vi "Read Config.vi"(8 "error in (no error)":errorcluster, 11 "Path":path) -> (0 "error out":errorcluster, 2 "Config":T1, 3 "File Created?":bool)   [LabVIEW 2020, in "VI Properties Editor.lvlib"]
doc: "Reads a config file located at <B>Path</B>."
uses:
  VI Properties Editor.lvlib
  CTLs/Config.ctl
  CTLs/Filter Info.ctl
  CTLs/Filter Column.ctl
  CTLs/Filter Type.ctl
  CTLs/Config Key.ctl
  9b94a6d9-a102-4d4c-a75a-250a13817fae.vi
  <vilib>/Utility/config.llb/Read Key (U32).vi
  <vilib>/Utility/config.llb/Read Key (String).vi
  <vilib>/Utility/config.llb/Read Key (Boolean).vi
  <vilib>/Utility/config.llb/Read Key (I32).vi
  <vilib>/Utility/config.llb/NI_LVConfig.lvlib
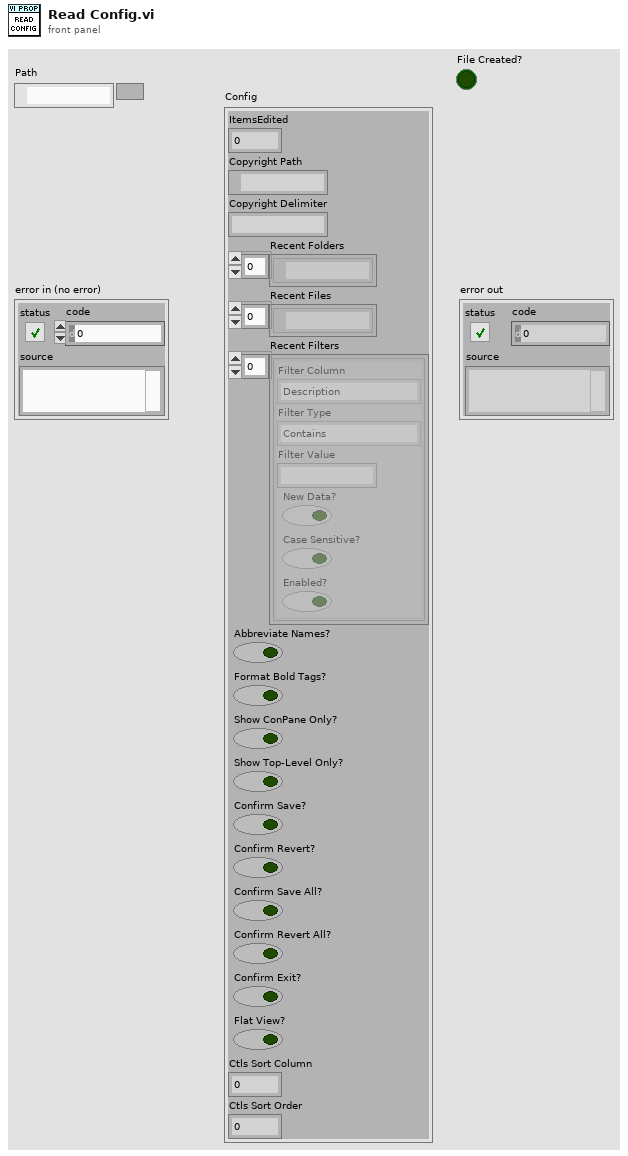
[diagram p1: front panel]
types:
  T1 = typedef "VI Properties Editor.lvlib/Config.ctl" = cluster{"ItemsEdited":u32, "Copyright Path":path, "Copyright Delimiter":string, "Recent Folders":path[], "Recent Files":path[], "Recent Filters":T2[], "Abbreviate Names?":bool, "Format Bold Tags?":bool, "Show ConPane Only?":bool, "Show Top-Level Only?":bool, "Confirm Save?":bool, "Confirm Revert?":bool, "Confirm Save All?":bool, "Confirm Revert All?":bool, "Confirm Exit?":bool, "Flat View?":bool, "Ctls Sort Column":i32, "Ctls Sort Order":i32}
  T2 = typedef "VI Properties Editor.lvlib/Filter Info.ctl" = cluster{"Filter Column":T3, "Filter Type":T4, "Filter Value":string, "New Data?":bool, "Case Sensitive?":bool, "Enabled?":bool}
  T3 = typedef "VI Properties Editor.lvlib/Filter Column.ctl" = enum16{"Name", "Path", "Type", "Window Title", "Description", "Help Path", "Help Tag", "Custom Title?", "Reentrancy", "Inlined?", "Help URL", "Help Type", "Allow Debugging?", "Auto Error Handling?", "Run When Opened?", "Suspend When Called?", "Priority", "Preferred Exec Sytem", "Control Label", "Control Caption", "Control Description", "Control Tip Strip"}
  T4 = typedef "VI Properties Editor.lvlib/Filter Type.ctl" = enum16{"Contains", "Equals", "Starts with", "Ends with", "Is empty", "Does not contain", "Does not equal", "Is not empty"}
  T5 = typedef "VI Properties Editor.lvlib/Config Key.ctl" = enum16{"ItemsEdited", "CopyrightPath", "CopyrightDelimiter", "RecentFolders", "RecentFiles", "RecentFilters", "AbbreviateNames", "ViewBold", "ShowCPCtlsOnly", "ShowTLCtlsOnly", "ConfirmSave", "ConfirmRevert", "ConfirmSaveAll", "ConfirmRevertAll", "ConfirmExit", "FlatView", "CtlsSortColumn", "CtlsSortOrder"}
  T6 = typedef "NI_LVConfig.lvlib/Config Data RefNum.ctl" = refnum<k1>
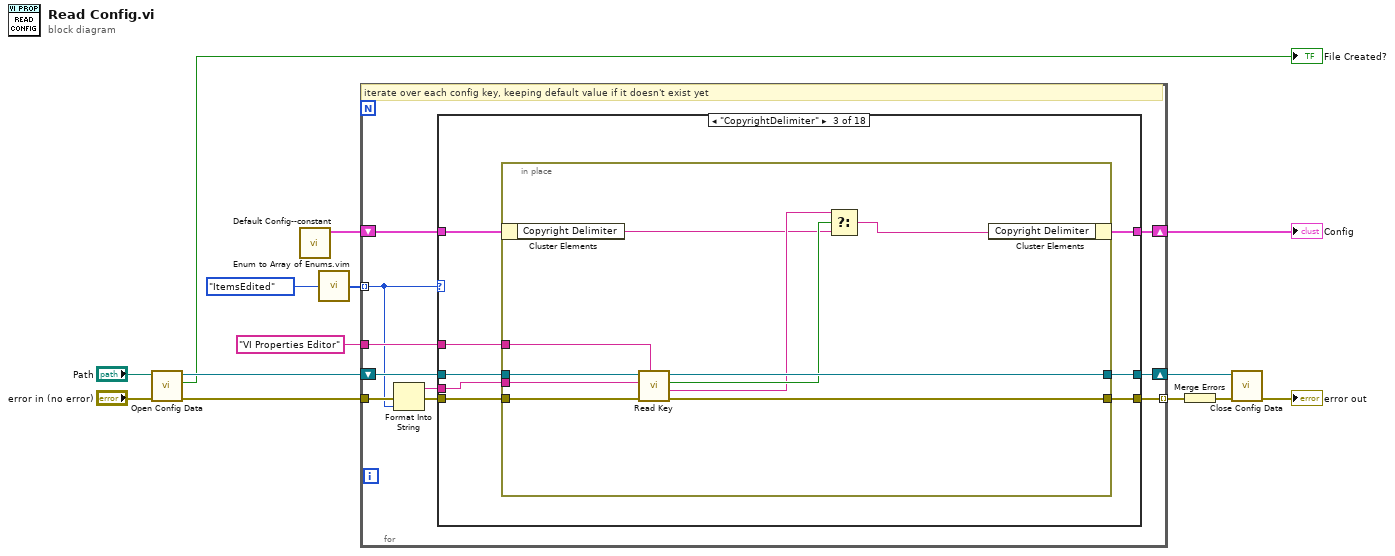
[diagram p0: block diagram]
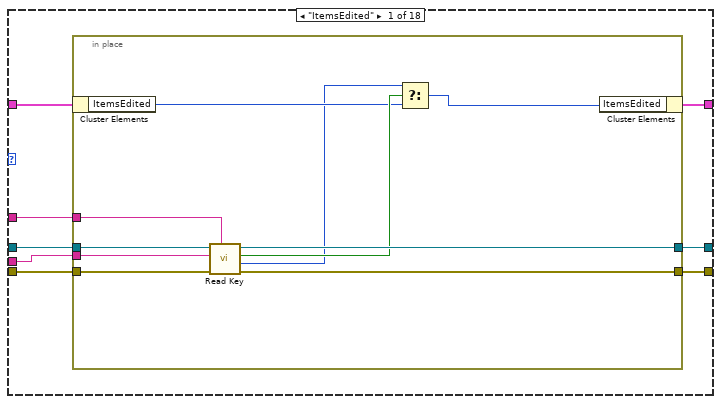
[diagram p2: hidden frame]
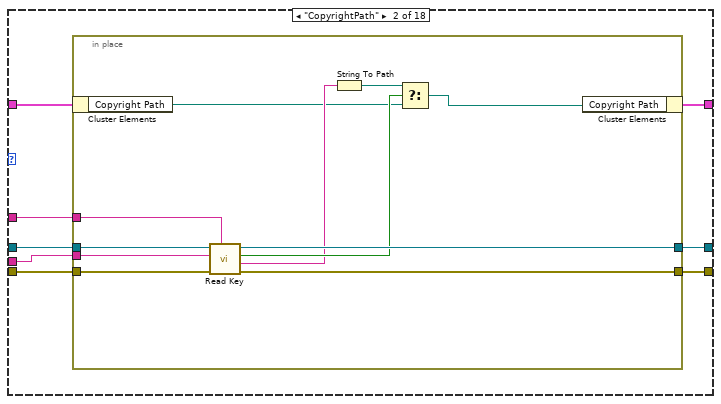
[diagram p3: hidden frame]
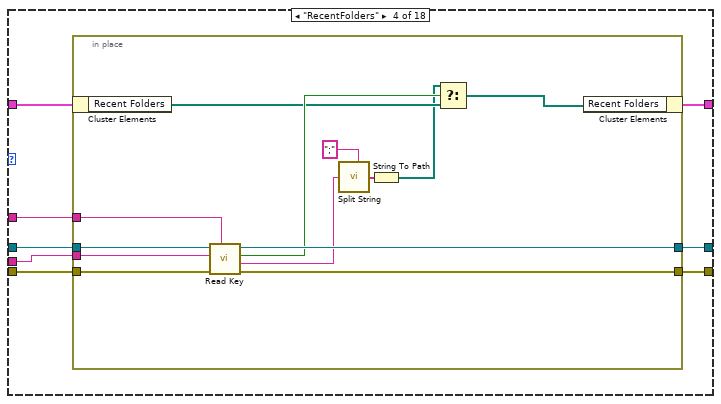
[diagram p4: hidden frame]
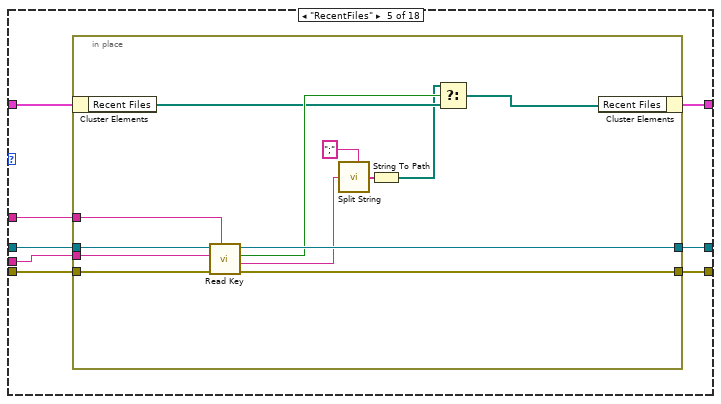
[diagram p5: hidden frame]
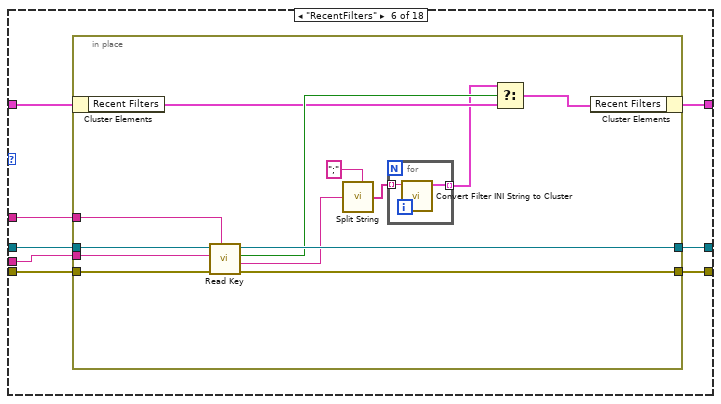
[diagram p6: hidden frame]
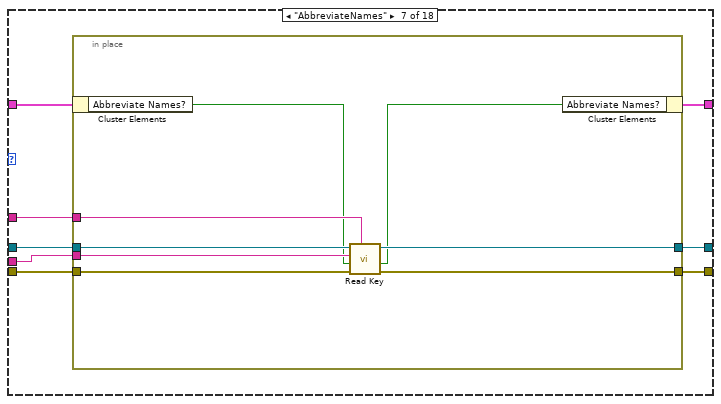
[diagram p7: hidden frame]
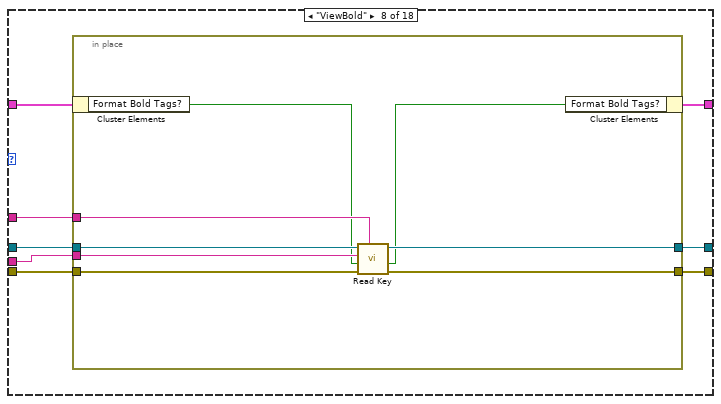
[diagram p8: hidden frame]
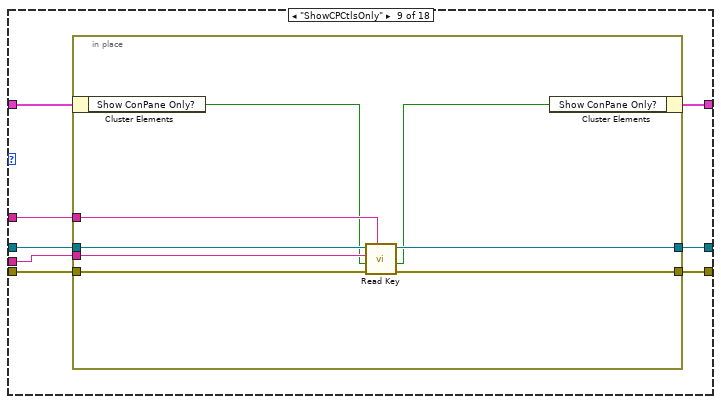
[diagram p9: hidden frame]
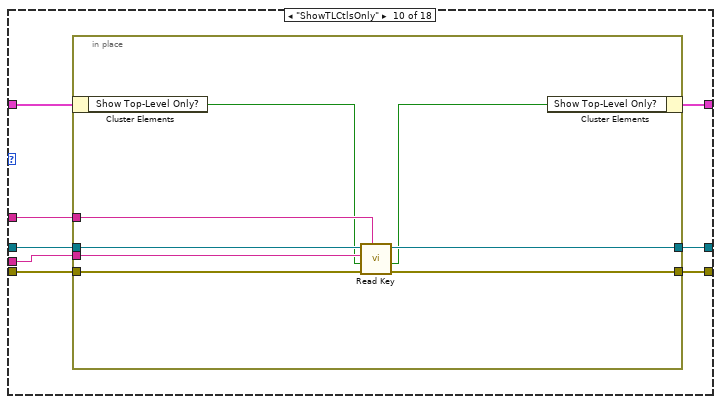
[diagram p10: hidden frame]
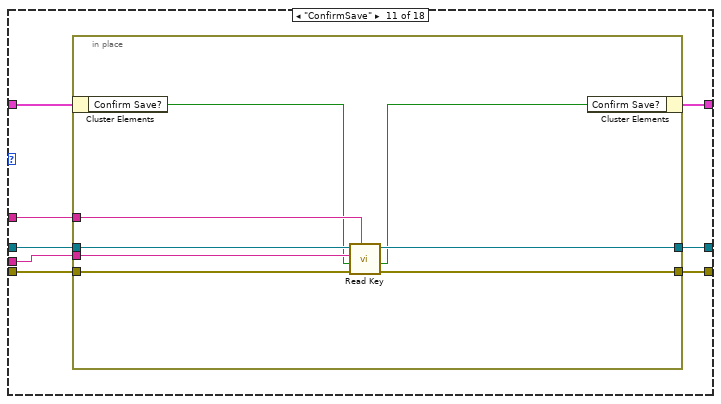
[diagram p11: hidden frame]
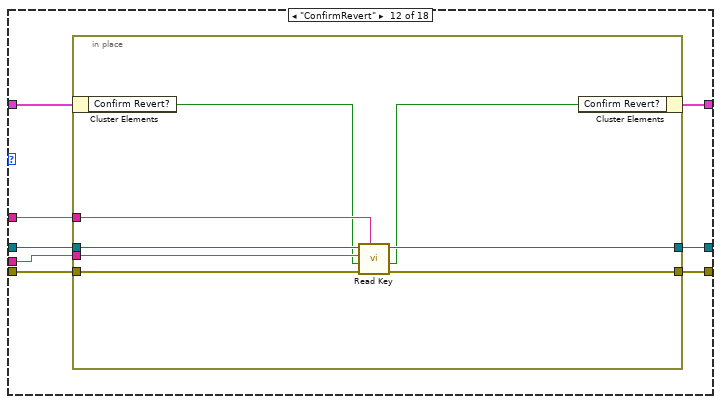
[diagram p12: hidden frame]
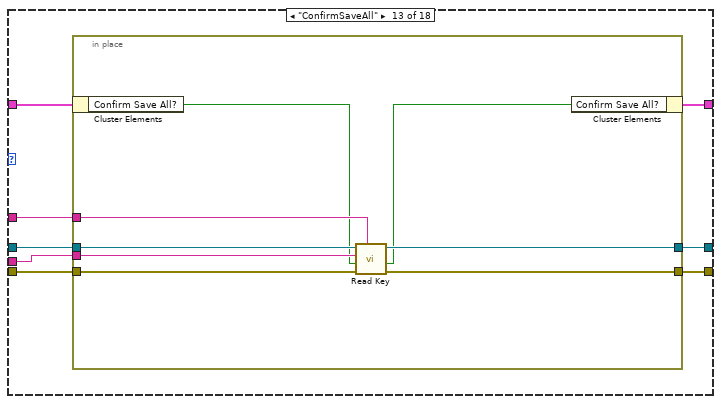
[diagram p13: hidden frame]
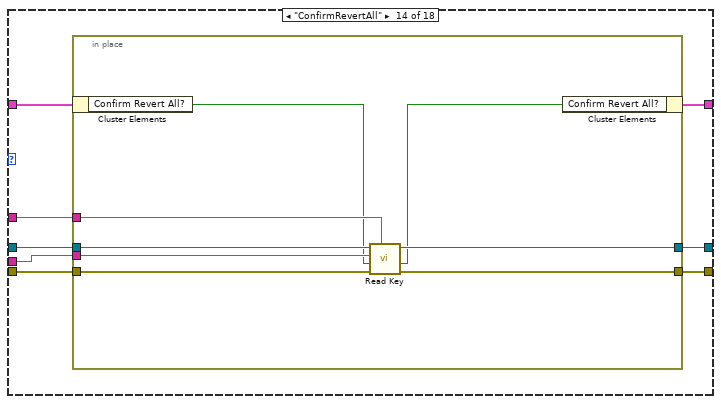
[diagram p14: hidden frame]
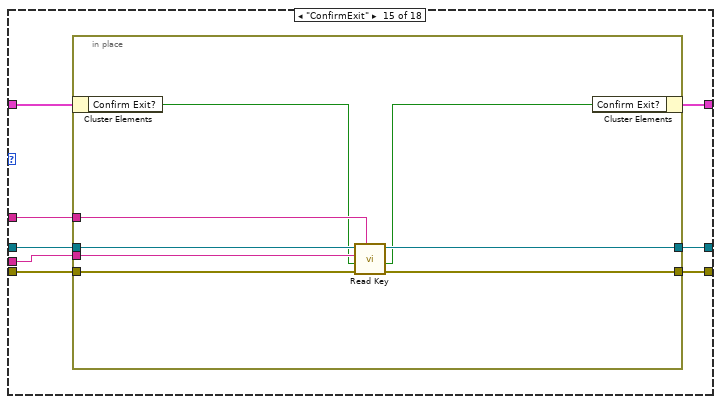
[diagram p15: hidden frame]
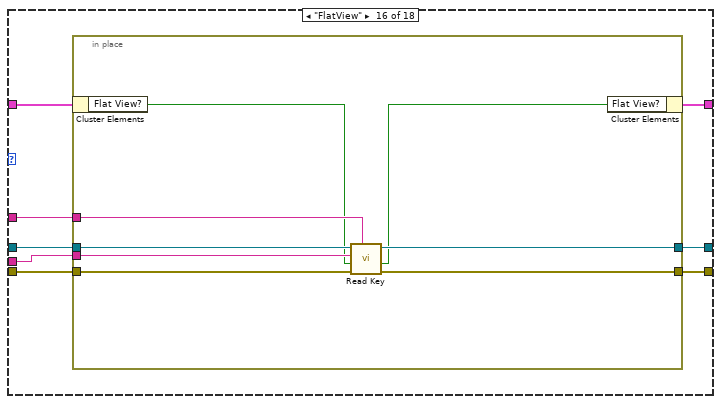
[diagram p16: hidden frame]
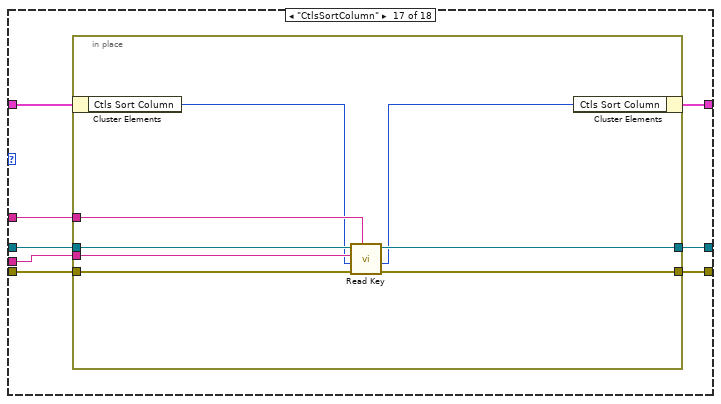
[diagram p17: hidden frame]
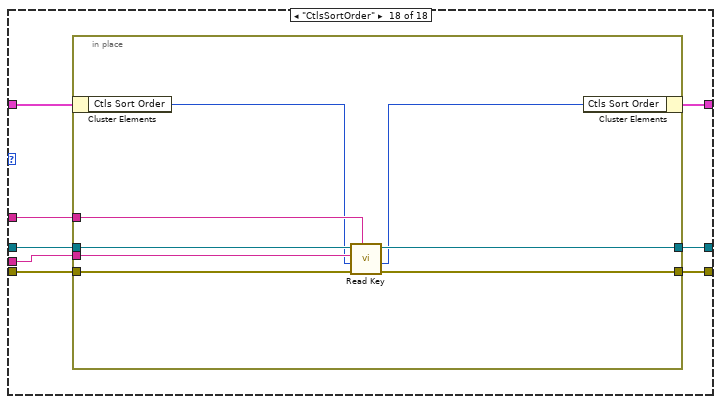
[diagram p18: hidden frame]
diagram:
  n1 = call <vilib>:"Open Config Data.vi"("error in (no error)"="error in (no error)", "configuration file path"="Path") -> ("error out"=w11:errorcluster, "file created?"=→"File Created?":bool, "refnum"=w14:T6)  [unwired: 7 in]
  n2 = call "Default Config--constant.vi"() -> ("Default Config"=w4:T1)  [unwired: 11 in]
  n3 = call "Enum to Array of Enums.vim"("enum"=Config_Key."ItemsEdited" ("Config Key")) -> ("array of enums"=w6:T5[])
  n4 = for {
    tunnel: w6 -> [w15] mode=indexing
    shift-right: [w18] -> w1
    shift-left: w4 -> [w21]
    tunnel: "VI Properties Editor" ("section") -> [w20]
    tunnel: [w23] -> w3 mode=indexing
    tunnel: w11 -> [w22]
    shift-right: [w16] -> w2
    shift-left: w14 -> [w17]
    # "iterate over each config key, keeping default value if it doesn't exist yet"
    n5 = Format Into String(error in=w22, w15) -> (resulting string=w19:string, error out=w24:errorcluster)  [unwired: 2 in]
    n6 = case shown="\"CopyrightDelimiter\"" w15 {
      tunnel: w21 -> [w28 w46 w65 w83 w104 w125 w148 w164 w180 w196 w212 w228 w244 w260 w276 w292 w308 w324]
      tunnel: w20 -> [w29 w47 w66 w84 w105 w126 w149 w165 w181 w197 w213 w229 w245 w261 w277 w293 w309 w325]
      tunnel: w19 -> [w30 w48 w67 w85 w106 w127 w150 w166 w182 w198 w214 w230 w246 w262 w278 w294 w310 w326]
      tunnel: w24 -> [w32 w50 w69 w87 w108 w129 w152 w168 w184 w200 w216 w232 w248 w264 w280 w296 w312 w328]
      tunnel: [w31 w49 w68 w86 w107 w128 w151 w167 w183 w199 w215 w231 w247 w263 w279 w295 w311 w327] -> w23
      tunnel: [w27 w45 w64 w82 w103 w124 w147 w163 w179 w195 w211 w227 w243 w259 w275 w291 w307 w323] -> w18
      tunnel: w17 -> [w26 w44 w63 w81 w102 w123 w146 w162 w178 w194 w210 w226 w242 w258 w274 w290 w306 w322]
      tunnel: [w25 w43 w62 w80 w101 w122 w145 w161 w177 w193 w209 w225 w241 w257 w273 w289 w305 w321] -> w16
      frame "ItemsEdited" {
        n7 = in-place {
          in-place-border: w30 -> [w39]
          in-place-border: w32 -> [w42]
          in-place-border: w29 -> [w38]
          in-place-border: [w41] -> w31
          in-place-border: w26 -> [w34]
          in-place-border: [w40] -> w25
          n8 = in-place-cluster #1(w28) -> ("ItemsEdited"=w36:u32)
          n9 = call-poly <vilib>:"Read Key.vi"("section"=w38, "error in (no error)"=w42, "key"=w39, "refnum"=w34) -> ("error out"=w41:errorcluster, "value"=w33:u32, "found?"=w37:bool, "refnum out"=w40:T6)  [unwired: 4 in]
          n10 = Select(t=w33, s=w37, f=w36) -> (s? t:f=w35:u32)
          n11 = in-place-cluster #1("ItemsEdited"=w35) -> (w27:T1)
        }
      }
      frame "CopyrightPath" {
        n12 = in-place {
          in-place-border: w48 -> [w58]
          in-place-border: w50 -> [w61]
          in-place-border: w47 -> [w57]
          in-place-border: [w60] -> w49
          in-place-border: w44 -> [w51]
          in-place-border: [w59] -> w43
          n13 = in-place-cluster #2(w46) -> ("Copyright Path"=w53:path)
          n14 = call-poly <vilib>:"Read Key.vi"("section"=w57, "error in (no error)"=w61, "key"=w58, "refnum"=w51) -> ("error out"=w60:errorcluster, "value"=w54:string, "found?"=w56:bool, "refnum out"=w59:T6)  [unwired: 4 in]
          n15 = String To Path(string=w54) -> (path=w55:path)
          n16 = Select(t=w55, s=w56, f=w53) -> (s? t:f=w52:path)
          n17 = in-place-cluster #2("Copyright Path"=w52) -> (w45:T1)
        }
      }
      frame "CopyrightDelimiter" {
        n18 = in-place {
          in-place-border: w67 -> [w76]
          in-place-border: w69 -> [w79]
          in-place-border: w66 -> [w75]
          in-place-border: [w78] -> w68
          in-place-border: w63 -> [w70]
          in-place-border: [w77] -> w62
          n19 = in-place-cluster #3(w65) -> ("Copyright Delimiter"=w72:string)
          n20 = call-poly <vilib>:"Read Key.vi"("section"=w75, "error in (no error)"=w79, "key"=w76, "refnum"=w70) -> ("error out"=w78:errorcluster, "value"=w73:string, "found?"=w74:bool, "refnum out"=w77:T6)  [unwired: 4 in]
          n21 = Select(t=w73, s=w74, f=w72) -> (s? t:f=w71:string)
          n22 = in-place-cluster #3("Copyright Delimiter"=w71) -> (w64:T1)
        }
      }
      frame "RecentFolders" {
        n23 = in-place {
          in-place-border: w85 -> [w97]
          in-place-border: w87 -> [w100]
          in-place-border: w84 -> [w96]
          in-place-border: [w99] -> w86
          in-place-border: w81 -> [w88]
          in-place-border: [w98] -> w80
          n24 = in-place-cluster #4(w83) -> ("Recent Folders"=w94:path[])
          n25 = call-poly <vilib>:"Read Key.vi"("section"=w96, "error in (no error)"=w100, "key"=w97, "refnum"=w88) -> ("error out"=w99:errorcluster, "value"=w90:string, "found?"=w95:bool, "refnum out"=w98:T6)  [unwired: 4 in]
          n26 = call <vilib>:"Split String.vi"("Split Pattern"=";", "Input String"=w90) -> ("Split String"=w92:string[])  [unwired: 5 in]
          n27 = String To Path(string=w92) -> (path=w89:path[])
          n28 = Select(t=w89, s=w95, f=w94) -> (s? t:f=w93:path[])
          n29 = in-place-cluster #4("Recent Folders"=w93) -> (w82:T1)
        }
      }
      frame "RecentFiles" {
        n30 = in-place {
          in-place-border: w106 -> [w118]
          in-place-border: w108 -> [w121]
          in-place-border: w105 -> [w117]
          in-place-border: [w120] -> w107
          in-place-border: w102 -> [w109]
          in-place-border: [w119] -> w101
          n31 = in-place-cluster #5(w104) -> ("Recent Files"=w115:path[])
          n32 = call-poly <vilib>:"Read Key.vi"("section"=w117, "error in (no error)"=w121, "key"=w118, "refnum"=w109) -> ("error out"=w120:errorcluster, "value"=w111:string, "found?"=w116:bool, "refnum out"=w119:T6)  [unwired: 4 in]
          n33 = call <vilib>:"Split String.vi"("Split Pattern"=";", "Input String"=w111) -> ("Split String"=w113:string[])  [unwired: 5 in]
          n34 = String To Path(string=w113) -> (path=w110:path[])
          n35 = Select(t=w110, s=w116, f=w115) -> (s? t:f=w114:path[])
          n36 = in-place-cluster #5("Recent Files"=w114) -> (w103:T1)
        }
      }
      frame "RecentFilters" {
        n37 = in-place {
          in-place-border: w127 -> [w139]
          in-place-border: w129 -> [w142]
          in-place-border: w126 -> [w138]
          in-place-border: [w141] -> w128
          in-place-border: w123 -> [w130]
          in-place-border: [w140] -> w122
          n38 = in-place-cluster #6(w125) -> ("Recent Filters"=w136:T2[])
          n39 = call-poly <vilib>:"Read Key.vi"("section"=w138, "error in (no error)"=w142, "key"=w139, "refnum"=w130) -> ("error out"=w141:errorcluster, "value"=w132:string, "found?"=w137:bool, "refnum out"=w140:T6)  [unwired: 4 in]
          n40 = call <vilib>:"Split String.vi"("Split Pattern"=";", "Input String"=w132) -> ("Split String"=w133:string[])  [unwired: 5 in]
          n41 = for {
            tunnel: w133 -> [w144] mode=indexing
            tunnel: [w143] -> w131 mode=indexing
            n42 = call "Convert Filter INI String to Cluster.vi"("INI String"=w144) -> ("Filter Info"=w143:T2)  [unwired: 10 in]
          }
          n43 = Select(t=w131, s=w137, f=w136) -> (s? t:f=w135:T2[])
          n44 = in-place-cluster #6("Recent Filters"=w135) -> (w124:T1)
        }
      }
      frame "AbbreviateNames" {
        n45 = in-place {
          in-place-border: w150 -> [w157]
          in-place-border: w152 -> [w160]
          in-place-border: w149 -> [w156]
          in-place-border: [w159] -> w151
          in-place-border: w146 -> [w155]
          in-place-border: [w158] -> w145
          n46 = in-place-cluster #7(w148) -> ("Abbreviate Names?"=w154:bool)
          n47 = call-poly <vilib>:"Read Key.vi"("section"=w156, "error in (no error)"=w160, "default value"=w154, "key"=w157, "refnum"=w155) -> ("error out"=w159:errorcluster, "value"=w153:bool, "refnum out"=w158:T6)  [unwired: 3 in, 1 out]
          n48 = in-place-cluster #7("Abbreviate Names?"=w153) -> (w147:T1)
        }
      }
      frame "ViewBold" {
        n49 = in-place {
          in-place-border: w166 -> [w173]
          in-place-border: w168 -> [w176]
          in-place-border: w165 -> [w172]
          in-place-border: [w175] -> w167
          in-place-border: w162 -> [w171]
          in-place-border: [w174] -> w161
          n50 = in-place-cluster #8(w164) -> ("Format Bold Tags?"=w170:bool)
          n51 = call-poly <vilib>:"Read Key.vi"("section"=w172, "error in (no error)"=w176, "default value"=w170, "key"=w173, "refnum"=w171) -> ("error out"=w175:errorcluster, "value"=w169:bool, "refnum out"=w174:T6)  [unwired: 3 in, 1 out]
          n52 = in-place-cluster #8("Format Bold Tags?"=w169) -> (w163:T1)
        }
      }
      frame "ShowCPCtlsOnly" {
        n53 = in-place {
          in-place-border: w182 -> [w189]
          in-place-border: w184 -> [w192]
          in-place-border: w181 -> [w188]
          in-place-border: [w191] -> w183
          in-place-border: w178 -> [w187]
          in-place-border: [w190] -> w177
          n54 = in-place-cluster #9(w180) -> ("Show ConPane Only?"=w186:bool)
          n55 = call-poly <vilib>:"Read Key.vi"("section"=w188, "error in (no error)"=w192, "default value"=w186, "key"=w189, "refnum"=w187) -> ("error out"=w191:errorcluster, "value"=w185:bool, "refnum out"=w190:T6)  [unwired: 3 in, 1 out]
          n56 = in-place-cluster #9("Show ConPane Only?"=w185) -> (w179:T1)
        }
      }
      frame "ShowTLCtlsOnly" {
        n57 = in-place {
          in-place-border: w198 -> [w205]
          in-place-border: w200 -> [w208]
          in-place-border: w197 -> [w204]
          in-place-border: [w207] -> w199
          in-place-border: w194 -> [w203]
          in-place-border: [w206] -> w193
          n58 = in-place-cluster #10(w196) -> ("Show Top-Level Only?"=w202:bool)
          n59 = call-poly <vilib>:"Read Key.vi"("section"=w204, "error in (no error)"=w208, "default value"=w202, "key"=w205, "refnum"=w203) -> ("error out"=w207:errorcluster, "value"=w201:bool, "refnum out"=w206:T6)  [unwired: 3 in, 1 out]
          n60 = in-place-cluster #10("Show Top-Level Only?"=w201) -> (w195:T1)
        }
      }
      frame "ConfirmSave" {
        n61 = in-place {
          in-place-border: w214 -> [w221]
          in-place-border: w216 -> [w224]
          in-place-border: w213 -> [w220]
          in-place-border: [w223] -> w215
          in-place-border: w210 -> [w219]
          in-place-border: [w222] -> w209
          n62 = in-place-cluster #11(w212) -> ("Confirm Save?"=w218:bool)
          n63 = call-poly <vilib>:"Read Key.vi"("section"=w220, "error in (no error)"=w224, "default value"=w218, "key"=w221, "refnum"=w219) -> ("error out"=w223:errorcluster, "value"=w217:bool, "refnum out"=w222:T6)  [unwired: 3 in, 1 out]
          n64 = in-place-cluster #11("Confirm Save?"=w217) -> (w211:T1)
        }
      }
      frame "ConfirmRevert" {
        n65 = in-place {
          in-place-border: w230 -> [w237]
          in-place-border: w232 -> [w240]
          in-place-border: w229 -> [w236]
          in-place-border: [w239] -> w231
          in-place-border: w226 -> [w235]
          in-place-border: [w238] -> w225
          n66 = in-place-cluster #12(w228) -> ("Confirm Revert?"=w234:bool)
          n67 = call-poly <vilib>:"Read Key.vi"("section"=w236, "error in (no error)"=w240, "default value"=w234, "key"=w237, "refnum"=w235) -> ("error out"=w239:errorcluster, "value"=w233:bool, "refnum out"=w238:T6)  [unwired: 3 in, 1 out]
          n68 = in-place-cluster #12("Confirm Revert?"=w233) -> (w227:T1)
        }
      }
      frame "ConfirmSaveAll" {
        n69 = in-place {
          in-place-border: w246 -> [w253]
          in-place-border: w248 -> [w256]
          in-place-border: w245 -> [w252]
          in-place-border: [w255] -> w247
          in-place-border: w242 -> [w251]
          in-place-border: [w254] -> w241
          n70 = in-place-cluster #13(w244) -> ("Confirm Save All?"=w250:bool)
          n71 = call-poly <vilib>:"Read Key.vi"("section"=w252, "error in (no error)"=w256, "default value"=w250, "key"=w253, "refnum"=w251) -> ("error out"=w255:errorcluster, "value"=w249:bool, "refnum out"=w254:T6)  [unwired: 3 in, 1 out]
          n72 = in-place-cluster #13("Confirm Save All?"=w249) -> (w243:T1)
        }
      }
      frame "ConfirmRevertAll" {
        n73 = in-place {
          in-place-border: w262 -> [w269]
          in-place-border: w264 -> [w272]
          in-place-border: w261 -> [w268]
          in-place-border: [w271] -> w263
          in-place-border: w258 -> [w267]
          in-place-border: [w270] -> w257
          n74 = in-place-cluster #14(w260) -> ("Confirm Revert All?"=w266:bool)
          n75 = call-poly <vilib>:"Read Key.vi"("section"=w268, "error in (no error)"=w272, "default value"=w266, "key"=w269, "refnum"=w267) -> ("error out"=w271:errorcluster, "value"=w265:bool, "refnum out"=w270:T6)  [unwired: 3 in, 1 out]
          n76 = in-place-cluster #14("Confirm Revert All?"=w265) -> (w259:T1)
        }
      }
      frame "ConfirmExit" {
        n77 = in-place {
          in-place-border: w278 -> [w285]
          in-place-border: w280 -> [w288]
          in-place-border: w277 -> [w284]
          in-place-border: [w287] -> w279
          in-place-border: w274 -> [w283]
          in-place-border: [w286] -> w273
          n78 = in-place-cluster #15(w276) -> ("Confirm Exit?"=w282:bool)
          n79 = call-poly <vilib>:"Read Key.vi"("section"=w284, "error in (no error)"=w288, "default value"=w282, "key"=w285, "refnum"=w283) -> ("error out"=w287:errorcluster, "value"=w281:bool, "refnum out"=w286:T6)  [unwired: 3 in, 1 out]
          n80 = in-place-cluster #15("Confirm Exit?"=w281) -> (w275:T1)
        }
      }
      frame "FlatView" {
        n81 = in-place {
          in-place-border: w294 -> [w301]
          in-place-border: w296 -> [w304]
          in-place-border: w293 -> [w300]
          in-place-border: [w303] -> w295
          in-place-border: w290 -> [w299]
          in-place-border: [w302] -> w289
          n82 = in-place-cluster #16(w292) -> ("Flat View?"=w298:bool)
          n83 = call-poly <vilib>:"Read Key.vi"("section"=w300, "error in (no error)"=w304, "default value"=w298, "key"=w301, "refnum"=w299) -> ("error out"=w303:errorcluster, "value"=w297:bool, "refnum out"=w302:T6)  [unwired: 3 in, 1 out]
          n84 = in-place-cluster #16("Flat View?"=w297) -> (w291:T1)
        }
      }
      frame "CtlsSortColumn" {
        n85 = in-place {
          in-place-border: w310 -> [w317]
          in-place-border: w312 -> [w320]
          in-place-border: w309 -> [w316]
          in-place-border: [w319] -> w311
          in-place-border: w306 -> [w315]
          in-place-border: [w318] -> w305
          n86 = in-place-cluster #17(w308) -> ("Ctls Sort Column"=w314:i32)
          n87 = call-poly <vilib>:"Read Key.vi"("section"=w316, "error in (no error)"=w320, "default value"=w314, "key"=w317, "refnum"=w315) -> ("error out"=w319:errorcluster, "value"=w313:i32, "refnum out"=w318:T6)  [unwired: 3 in, 1 out]
          n88 = in-place-cluster #17("Ctls Sort Column"=w313) -> (w307:T1)
        }
      }
      frame "CtlsSortOrder" {
        n89 = in-place {
          in-place-border: w326 -> [w333]
          in-place-border: w328 -> [w336]
          in-place-border: w325 -> [w332]
          in-place-border: [w335] -> w327
          in-place-border: w322 -> [w331]
          in-place-border: [w334] -> w321
          n90 = in-place-cluster #18(w324) -> ("Ctls Sort Order"=w330:i32)
          n91 = call-poly <vilib>:"Read Key.vi"("section"=w332, "error in (no error)"=w336, "default value"=w330, "key"=w333, "refnum"=w331) -> ("error out"=w335:errorcluster, "value"=w329:i32, "refnum out"=w334:T6)  [unwired: 3 in, 1 out]
          n92 = in-place-cluster #18("Ctls Sort Order"=w329) -> (w323:T1)
        }
      }
    }
  }
  "Config" <- w1
  n93 = Merge Errors(w3) -> (w10:errorcluster)
  n94 = call <vilib>:"Close Config Data.vi"("error in (no error)"=w10, "refnum"=w2) -> ("error out"=→"error out":errorcluster)  [unwired: 8 in, 1 out]
